vi "SJ_ODE_RHS_PRESS.vi"(2 "data":T1, 3 "t":dbl, 4 "x":dbl[](array[numeric])) -> (0 "error out":errorcluster, 1 "f(x,t)":dbl[](array[numeric]))   [LabVIEW 2012]
doc: "This template is the starting point for creating a function that is the right-hand-side of an ordinary differential equaltion to be passed to the ODE Solver.vi."
uses:
  <vilib>/gmath/NumericalOptimization/objective function data.ctl
  SJ_ODE_Data.ctl
  Utilities/fluid_properties/fluid_types.ctl
  Model.ctl
  Utilities/fluid_properties/fluid_properties.ctl
  <vilib>/gmath/NI_Gmath.lvlib
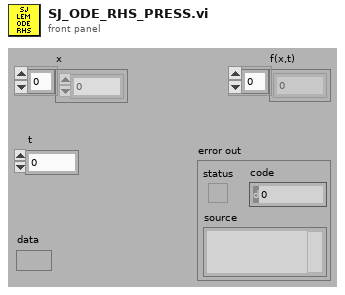
[diagram p1: front panel]
types:
  T1 = typedef "NI_Gmath.lvlib/objective function data.ctl" = variant
  T2 = typedef "SJ_ODE_Data.ctl" = cluster{"Fluid Properties":cluster{"Fluid":T3, "Temperature (K)":dbl, "Pressure (Pa)":dbl}, "SJ Geometry":cluster{"Do (mm)":dbl, "Ho (mm)":dbl, "Dc (mm)":dbl, "Hc (mm)":dbl}, "Solution Controls":cluster{"Simulation":enum16{"Asymmetric", "Sinusoidal"}, "Fixed Parameter":enum16{"Pressure", "Displacement"}, "Model":T4, "# time steps":i32, "# periods":i32, "Domain":enum16{"Time", "Frequency"}}, "Misc Data":cluster{"Amplitude Array":dbl[], "Freq jet":dbl, "Coefficients":dbl[]}, "Thermo and Transport Properties":T5, "LEM Output Data":cluster{"X":dbl[][], "times":dbl[], "|X|":dbl, "PA X":dbl}}
  T3 = typedef "fluid_types.ctl" = enum16{"Air", "Water"}
  T4 = typedef "Model.ctl" = enum16{"Tang", "Gallas", "Persoon"}
  T5 = typedef "fluid_properties.ctl" = cluster{"nu":dbl, "c":dbl, "Pr":dbl, "Cp":dbl, "Cv":dbl, "gamma":dbl, "mu":dbl, "rho":dbl}
  T6 = cluster{"Amplitude Array":dbl[], "Freq jet":dbl, "Coefficients":dbl[]}
  T7 = cluster{"Simulation":enum16{"Asymmetric", "Sinusoidal"}, "Fixed Parameter":enum16{"Pressure", "Displacement"}, "Model":T4, "# time steps":i32, "# periods":i32, "Domain":enum16{"Time", "Frequency"}}
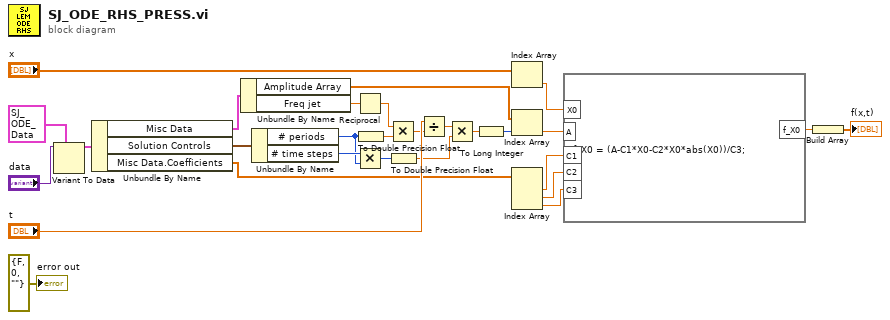
[diagram p0: block diagram]
diagram:
  n1 = Variant To Data(type=T2 {"Fluid Properties"={"Fluid"=enum."Air", "Temperature (K)"=0.0, "Pressure (Pa)"=0.0}, "SJ Geometry"={"Do (mm)"=0.0, "Ho (mm)"=0.0, "Dc (mm)"=0.0, "Hc (mm)"=0.0}, "Solution Controls"={"Simulation"=enum."Asymmetric", "Fixed Parameter"=enum."Pressure", "Model"=enum."Tang", "# time steps"=0, "# periods"=0, "Domain"=enum."Time"}, "Misc Data"={"Amplitude Array"=[], "Freq jet"=0.0, "Coefficients"=[]}, "Thermo and Transport Properties"={"nu"=0.0, "c"=0.0, "Pr"=0.0, "Cp"=0.0, "Cv"=0.0, "gamma"=0.0, "mu"=0.0, "rho"=0.0}, "LEM Output Data"={"X"=[], "times"=[], "|X|"=0.0, "PA X"=0.0}} ("ODE Data"), Variant="data") -> (data=w26:T2)  [unwired: 1 in, 1 out]
  n2 = Unbundle By Name(w26) -> ("Misc Data"=w20:T6, "Solution Controls"=w21:T7, "Misc Data.Coefficients"=w4:dbl[])
  n3 = Unbundle By Name(w20) -> ("Amplitude Array"=w18:dbl[], "Freq jet"=w16:dbl)
  n4 = Unbundle By Name(w21) -> ("# periods"=w6:i32, "# time steps"=w7:i32)
  n5 = Reciprocal(x=w16) -> (1/x=w15:dbl)
  n6 = Multiply(x=w7, y=w6) -> (x*y=w5:i32)
  n7 = To Double Precision Float(number=w6) -> (double precision float=w14:dbl)
  n8 = Multiply(x=w15, y=w14) -> (x*y=w12:dbl)
  n9 = To Double Precision Float(number=w5) -> (double precision float=w10:dbl)
  n10 = Divide(x="t", y=w12) -> (x/y=w11:dbl)
  n11 = Multiply(x=w11, y=w10) -> (x*y=w9:dbl)
  n12 = To Long Integer(number=w9) -> (32bit integer=w19:i32)
  n13 = Index Array(array="x") -> (element=w23:dbl)  [unwired: 1 in]
  n14 = Index Array(array=w18, index=w19) -> (element=w8:dbl)
  n15 = Index Array(array=w4) -> (element #1=w3:dbl, element #2=w2:dbl, element #3=w1:dbl)  [unwired: 3 in]
  n16 = formula code="f_X0 = (A-C1*X0-C2*X0*abs(X0))/C3;"("C1"=w3, "C2"=w2, "C3"=w1, "X0"=w23, "A"=w8) -> ("f_X0"=w22:dbl)
  n17 = Build Array(w22) -> (→"f(x,t)":dbl[])
  "error out" <- errorcluster {"status"=FALSE, "code"=0, "source"=""} ("error out")
